vi "getGainInUse.vi"(8 "error in (no error)":errorcluster, 11 "ZTAAC in":refnum<class "ZTAAC.lvclass">) -> (0 "error out":errorcluster, 2 "Gain in Use":dbl, 3 "ZTAAC out":refnum<class "ZTAAC.lvclass">)   [LabVIEW 2016, in "OfcFunc.lvlib" / "ZTAAC.lvclass"]
doc: "Get the gain value used in the Optimal Control. It is noted that the gain value in use might be different from the default gain value if the image quality is bad (Gain = 1)."
uses:
  ZTAAC.lvclass
  ZTAAC.lvclass/ZTAAC.ctl
  OptCtrl/OptCtrl.lvclass
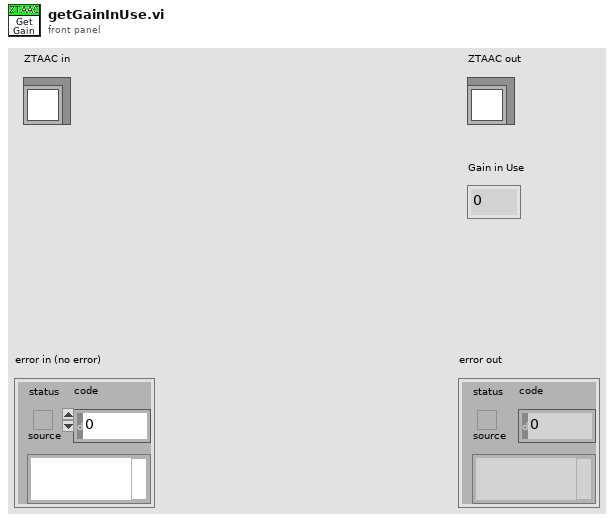
[diagram p1: front panel]
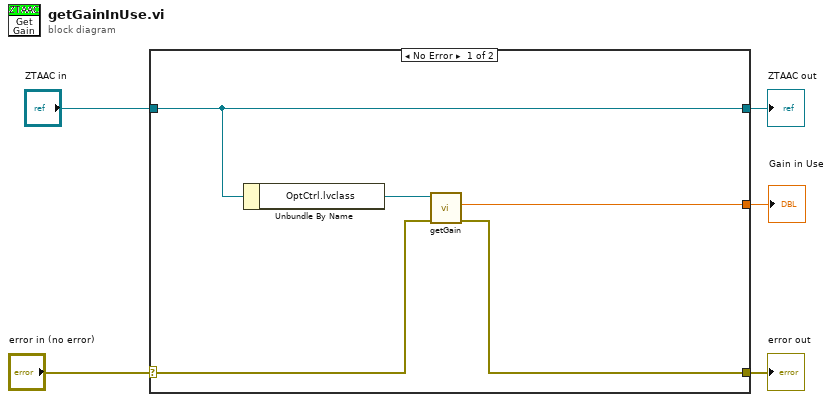
[diagram p0: block diagram]
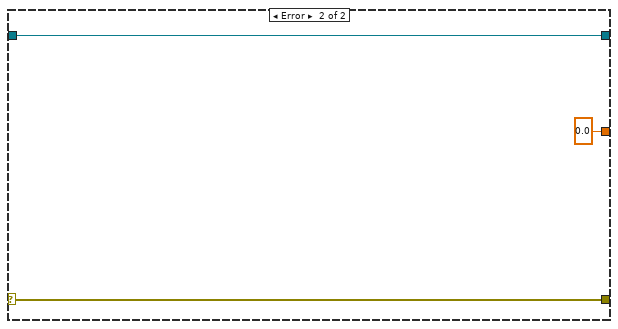
[diagram p2: hidden frame]
diagram:
  n1 = case shown="No Error" "error in (no error)" {
    selector: "error in (no error)" -> [w8 w13]
    tunnel: [w7 w13] -> w4
    tunnel: [w10 w12] -> w2
    tunnel: "ZTAAC in" -> [w10 w12]
    tunnel: [w6 0.0 ("Gain")] -> w1
    frame No Error {
      n2 = Unbundle By Name(w10) -> ("OptCtrl.lvclass"=w9:refnum<class "OptCtrl.lvclass">)
      n3 = call "getGain.vi"("error in (no error)"=w8, "OptCtrl in"=w9) -> ("error out"=w7:errorcluster, "Gain"=w6:dbl)  [unwired: 7 in, 1 out]
    }
    frame Error {
    }
  }
  "error out" <- w4
  "ZTAAC out" <- w2
  "Gain in Use" <- w1
